vi "PicoScope2000aExampleAWG.vi"() -> ()   [LabVIEW 2018]
uses:
  PS2000a.dll
panel:
  in  "Standard Waveform Settings":T1={"Start Frequency"=10000.0, "Stop Frequency"=10000.0, "Increment"=0.0, "Dwell Time (seconds)"=0.0} {"Stop Frequency" min=0.03 max=1000000.0; "Start Frequency" min=0.03 max=1000000.0}
  in  "Arbitrary Waveform Settings":T2 {"Index Mode" items=["Single", "Dual", "Quad"]}
  in  "Software \nTrigger":bool
  in  "Stop S/W \nTrigger":bool
  out "Arbitrary\nWaveform Graph":i16[](graph)
  in  "Update":bool
  in  "stop":bool
  in  "General AWG Settings":T3={"Peak-to-Peak Voltage (microvolts)"=2000000, "Offset Voltage (microvolts)"=1000000, "Wave Type"=1, "Sweep Type"=0, "Shots"=0, "Sweeps"=0, "Trigger Type"=0, "Trigger Source"=0, "Ext. Threshold (ADC count)"=0, "White Noise"=FALSE} {"Trigger Source" items=["None", "Scope Trigger", "Aux. In", "Ext. In", "Software Trigger"]; "Trigger Type" items=["Rising", "Falling", "Gate High", "Gate Low"]; "Sweep Type" items=["Up", "Down", "Up-Down", "Down-Up"]; "Wave Type" items=["Sine"=0, "Square"=1, "Triangle"=2, "Ramp Up"=3, "Ramp Down"=4, "DC"=8, "Arbitrary"=6]}
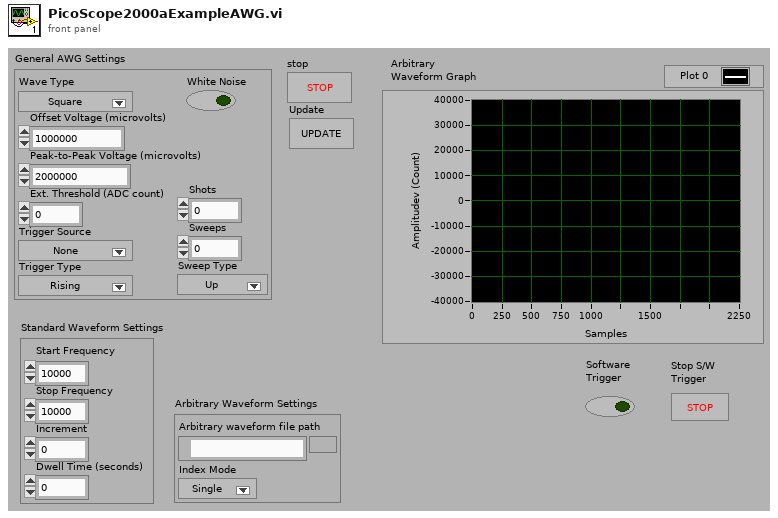
[diagram p1: front panel]
types:
  T1 = cluster{"Start Frequency":dbl, "Stop Frequency":dbl, "Increment":dbl, "Dwell Time (seconds)":dbl}
  T2 = cluster{"Arbirary waveform file path":path, "Index Mode":u32}
  T3 = cluster{"Peak-to-Peak Voltage (microvolts)":u32, "Offset Voltage (microvolts)":i32, "Wave Type":i16, "Sweep Type":i32, "Shots":u32, "Sweeps":u32, "Trigger Type":i32, "Trigger Source":i32, "Ext. Threshold (ADC count)":i16, "White Noise":bool}
  T4 = cluster{"Driver Version":string, "USB Version":string, "Hardware":string, "Variant":string, "Batch and Serial":string, "Cal Date":string, "Kernel Version":string, "Digital HW Version":string, "Analogue HW Version":string, "Firmware 1":string, "Firmware 2":string, "MSO":bool, "Number of Channels":i16}
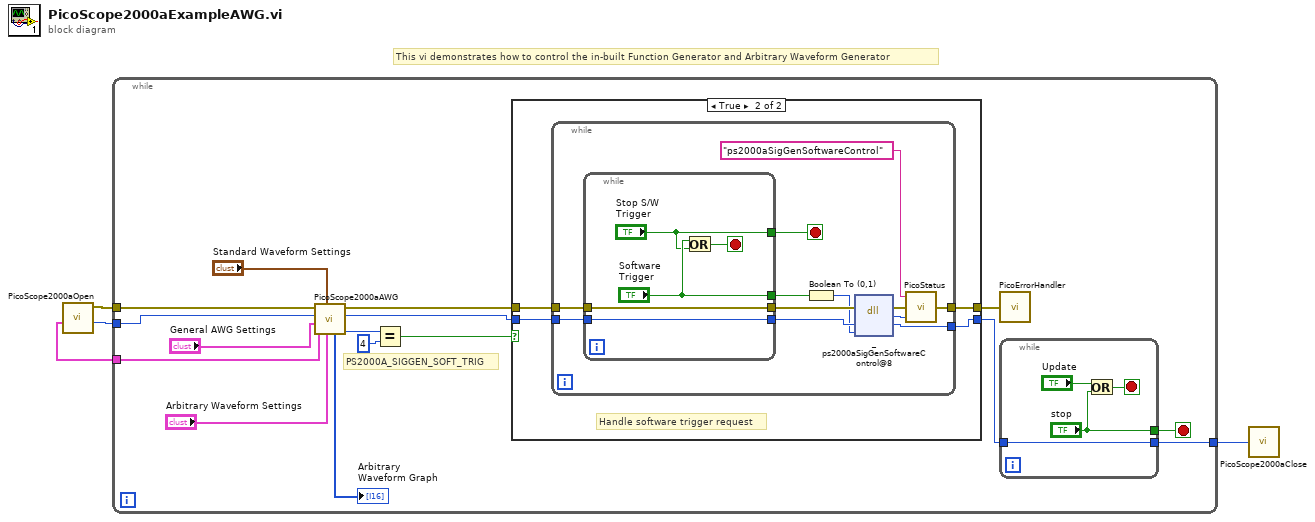
[diagram p0: block diagram]
diagram:
  # "This vi demonstrates how to control the in-built Function Generator and Arbitrary Waveform Generator"
  n1 = call "PicoScope2000aOpen.vi"() -> ("handle"=w3:i16, "error out"=w2:errorcluster, "Device Info"=w1:T4)  [unwired: 4 in, 1 out]
  n2 = while {
    tunnel: [w20] -> w4
    tunnel: w3 -> [w18]
    tunnel: w2 -> [w17]
    tunnel: w1 -> [w6]
    stop <- w16 stop-if-true
    # "PS2000A_SIGGEN_SOFT_TRIG"
    n3 = call "PicoScope2000aAWG.vi"("Arbitrary Waveform Settings"="Arbitrary Waveform Settings", "Standard Waveform Settings"="Standard Waveform Settings", "Device Info"=w6, "General AWG Settings"="General AWG Settings", "Handle In"=w18, "error in"=w17) -> ("triggerSource"=w9:i32, "Handle Out"=w11:i16, "error out"=w14:errorcluster, "Arbitrary\nWaveform Graph"=→"Arbitrary\nWaveform Graph":i16[])  [unwired: 2 in]
    n4 = Equal?(x=w9, y=4) -> (x = y?=w10:bool)
    n5 = case shown="True" w10 {
      tunnel: [w22 w24] -> w12
      tunnel: w14 -> [w22 w26]
      tunnel: [w21 w25] -> w13
      tunnel: w11 -> [w21 w23]
      frame False {
      }
      frame True {
        # "Handle software trigger request"
        n6 = while {
          tunnel: w26 -> [w37]
          tunnel: w23 -> [w36]
          tunnel: [w34] -> w25
          tunnel: [w27] -> w24
          stop <- w31 stop-if-true
          n7 = while {
            tunnel: [w43] -> w38
            tunnel: w37 -> [w43]
            tunnel: ["Software \nTrigger"] -> w33
            tunnel: w36 -> [w42]
            tunnel: [w42] -> w35
            tunnel: ["Stop S/W \nTrigger"] -> w31
            stop <- w39 stop-if-true
            n8 = Or(x="Software \nTrigger", y="Stop S/W \nTrigger") -> (x .or. y?=w39:bool)
          }
          n9 = Boolean To (0,1)(Boolean=w33) -> (0, 1=w32:i16)
          n10 = dll-call lib="ps2000a.dll" fn="_ps2000aSigGenSoftwareControl@8"(error in=w38, "handle"=w35, "state"=w32) -> (error out=w29:errorcluster, "PICO_STATUS"=w30:u32, "handle"=w34:i16)  [unwired: 3 in, 1 out]
          n11 = call "PicoStatus.vi"("PICO STATUS"=w30, "error in"=w29, "source"="ps2000aSigGenSoftwareControl") -> ("error out"=w27:errorcluster)
        }
      }
    }
    n12 = call "PicoErrorHandler.vi"("error in"=w12) -> ()  [unwired: 1 out]
    n13 = while {
      tunnel: [w47] -> w20
      tunnel: w13 -> [w47]
      tunnel: ["stop"] -> w16
      stop <- w46 stop-if-true
      n14 = Or(x="Update", y="stop") -> (x .or. y?=w46:bool)
    }
  }
  n15 = call "PicoScope2000aClose.vi"("handle"=w4) -> ()
